vi "Get Gripper Notifier.vi"() -> (3 "Notifier out":refnum<notifier>)   [LabVIEW 2014, in "Elevator System.lvlib"]
uses:
  Elevator System.lvlib
  Typedef/GripperNotifierType.ctl
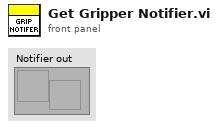
[diagram p1: front panel]
types:
  T1 = typedef "Elevator System.lvlib/GripperNotifierType.ctl" = cluster{"SP Left":dbl, "SP Right":dbl}
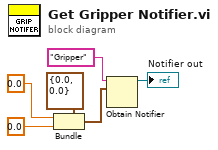
[diagram p0: block diagram]
diagram:
  n1 = Bundle(cluster=T1 {"SP Left"=0.0, "SP Right"=0.0}, "SP Left"=0.0 ("Setpoint"), "SP Right"=0.0 ("Setpoint")) -> (w6:T1)
  n2 = Obtain Notifier(name (unnamed)="Gripper", notification data type=w6) -> (notifier out=→"Notifier out":refnum<notifier>)  [unwired: 2 in, 2 out]
